vi "DriveWaitForManip.vi"(2 "Parameter String":string, 3 "Reinit":bool) -> (0 "Error Out":errorcluster, 1 "Increment":bool)   [LabVIEW 2019]
doc: "This VI pauses the drive sequencer until the manipulator sequencer has reached (or passed) the specified step.\n\nParameters:\nParam1: manipulator step to wait for"
uses:
  SafeParser_Integer.vi
  dscommands.vi
  autoninfo.vi
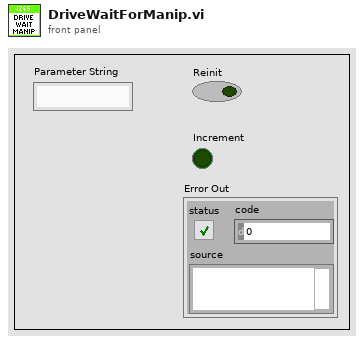
[diagram p1: front panel]
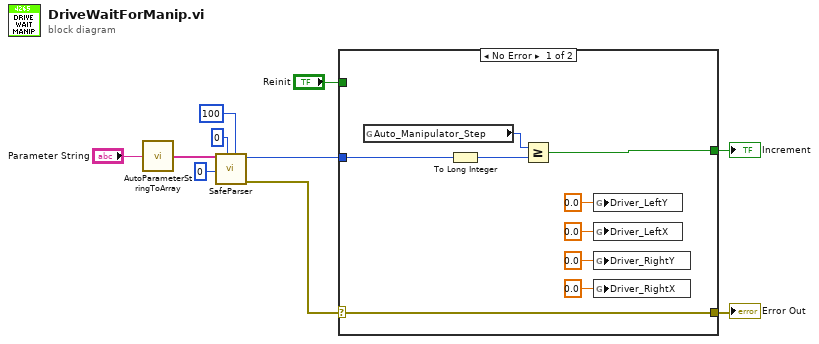
[diagram p0: block diagram]
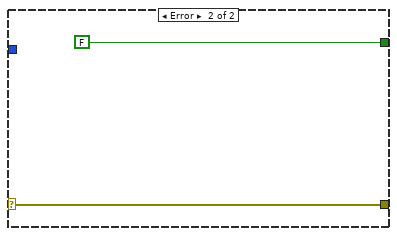
[diagram p2: hidden frame]
diagram:
  n1 = call "AutoParameterStringToArray.vi"("Parameter String"="Parameter String") -> ("Parsed Parameters"=w2:string[])
  n2 = call-poly "SafeParser.vi"("Maximum"=100, "Minimum"=0, "Array Index"=0 ("Parameter Index"), "String Array"=w2) -> ("Error Out"=w1:errorcluster, "Typecast  Value"=w6:i32)  [unwired: 6 in]
  n3 = case shown="No Error" w1 {
    selector: w1 -> [w15 w21]
    tunnel: [w11 FALSE] -> w10
    tunnel: "Reinit" -> [_ _]
    tunnel: [w15 w21] -> w8
    tunnel: w6 -> [w12 _]
    frame No Error {
      n4 = global read "autoninfo.vi" "Auto_Manipulator_Step"() -> (w14:i32)
      n5 = To Long Integer(number=w12) -> (32bit integer=w13:i32)
      n6 = Greater Or Equal?(x=w14, y=w13) -> (x >= y?=w11:bool)
      n7 = global write "dscommands.vi" "Driver_LeftY"(0.0 ("Driver_LeftY")) -> ()
      n8 = global write "dscommands.vi" "Driver_LeftX"(0.0 ("Driver_RightX")) -> ()
      n9 = global write "dscommands.vi" "Driver_RightY"(0.0 ("Driver_RightX")) -> ()
      n10 = global write "dscommands.vi" "Driver_RightX"(0.0 ("Driver_RightX")) -> ()
    }
    frame Error {
    }
  }
  "Increment" <- w10
  "Error Out" <- w8
